vi "UdpDataGlobal.vi"(0 "Position":dbl, 1 "Starting Position":dbl, 2 "Target Position":dbl, 3 "Force":dbl, 4 "TargetState":bool, 5 "RomState":T1, 6 "Time":dbl, 7 "Finished":bool, 8 "Flexion":bool, 9 "Trial Nr":i16, 12 "Action":T3) -> (23 "UDP Robot State":T2)   [LabVIEW 2015]
uses:
  UdpGlobalActions.ctl
  UDPRobotState.ctl
  All_In_One/States/ROM_States.ctl
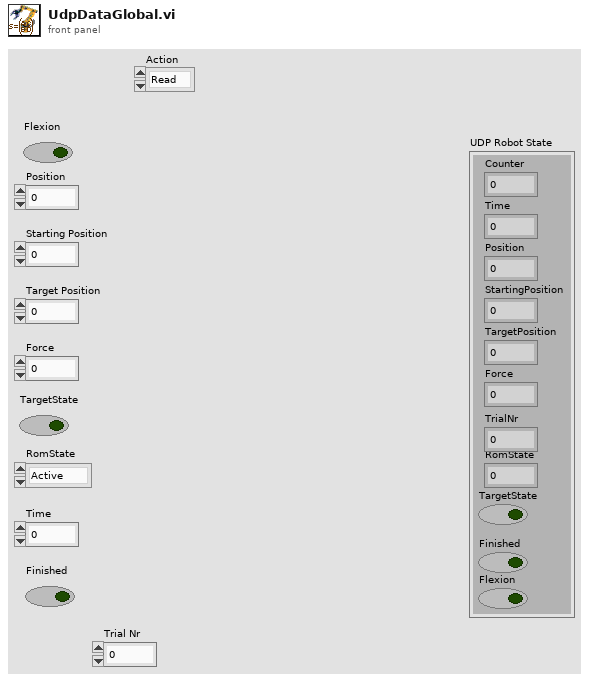
[diagram p1: front panel]
types:
  T1 = typedef "ROM_States.ctl" = enum8{"Active", "Passive", "AutomaticPassive"}
  T2 = typedef "UDPRobotState.ctl" = cluster{"Counter":u32, "Time":sgl, "Position":sgl, "StartingPosition":sgl, "TargetPosition":sgl, "Force":sgl, "TrialNr":u8, "RomState":u8, "TargetState":bool, "Finished":bool, "Flexion":bool}
  T3 = typedef "UdpGlobalActions.ctl" = enum16{"Read", "Write"}
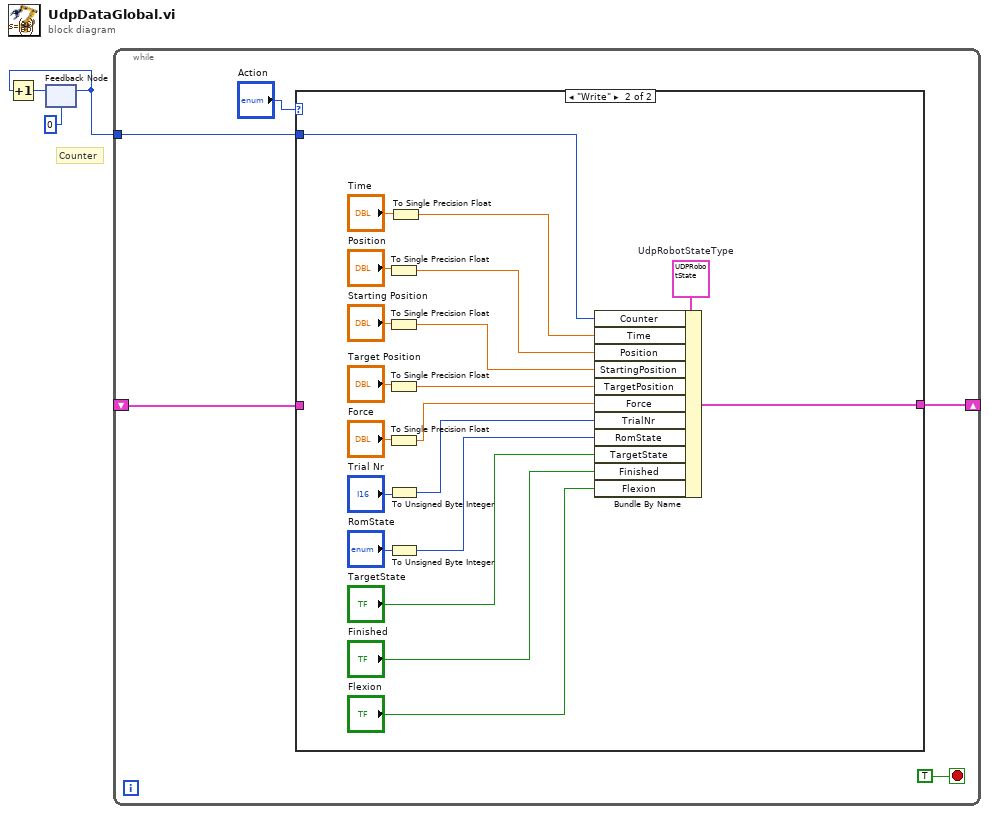
[diagram p0: block diagram]
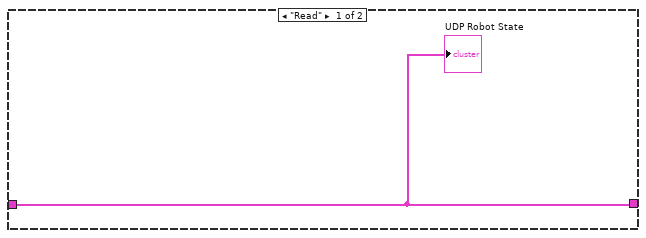
[diagram p2: hidden frame]
diagram:
  # "Counter"
  n1 = feedback #1(u32 0) -> (w1:u32)
  n2 = Increment(x=w1) -> (x+1=w3:u32)
  n3 = feedback-in #1(w3) -> ()
  n4 = while {
    shift-right: [w5] -> _
    shift-left: _ -> [w4]
    tunnel: w1 -> [w6]
    stop <- TRUE stop-if-true
    n5 = case shown="\"Write\"" "Action" {
      tunnel: w6 -> [_ w20]
      tunnel: [w9 w28] -> w5
      tunnel: w4 -> [w9 _]
      frame "Read" {
        "UDP Robot State" <- w9
      }
      frame "Write" {
        w29 = T2 {"Counter"=0, "Time"=0.0, "Position"=0.0, "StartingPosition"=0.0, "TargetPosition"=0.0, "Force"=0.0, "TrialNr"=0, "RomState"=0, "TargetState"=FALSE, "Finished"=FALSE, "Flexion"=FALSE}  # UdpRobotStateType
        n6 = To Single Precision Float(number="Position") -> (single precision float=w16:sgl)
        n7 = To Single Precision Float(number="Starting Position") -> (single precision float=w17:sgl)
        n8 = To Single Precision Float(number="Target Position") -> (single precision float=w18:sgl)
        n9 = To Single Precision Float(number="Force") -> (single precision float=w19:sgl)
        n10 = To Unsigned Byte Integer(number="Trial Nr") -> (unsigned 8bit integer=w10:u8)
        n11 = To Unsigned Byte Integer(number="RomState") -> (unsigned 8bit integer=w11:u8)
        n12 = To Single Precision Float(number="Time") -> (single precision float=w15:sgl)
        n13 = Bundle By Name(cluster=w29, "Counter"=w20, "Time"=w15, "Position"=w16, "StartingPosition"=w17, "TargetPosition"=w18, "Force"=w19, "TrialNr"=w10, "RomState"=w11, "TargetState"="TargetState", "Finished"="Finished", "Flexion"="Flexion") -> (w28:T2)
      }
    }
  }
